vi "HTS_GET_PMC_COMMANDS.vi"(8 "Error IN":errorcluster, 11 "VISA resource IN":refnum<visa-resource-name>="HTS") -> (0 "Error OUT":errorcluster, 2 "HTS_PMC_COMMANDS":T1, 3 "VISA resource OUT":refnum<visa-resource-name>)   [LabVIEW 2009]
uses:
  HTS_PMC_COMMAND_LIST.ctl
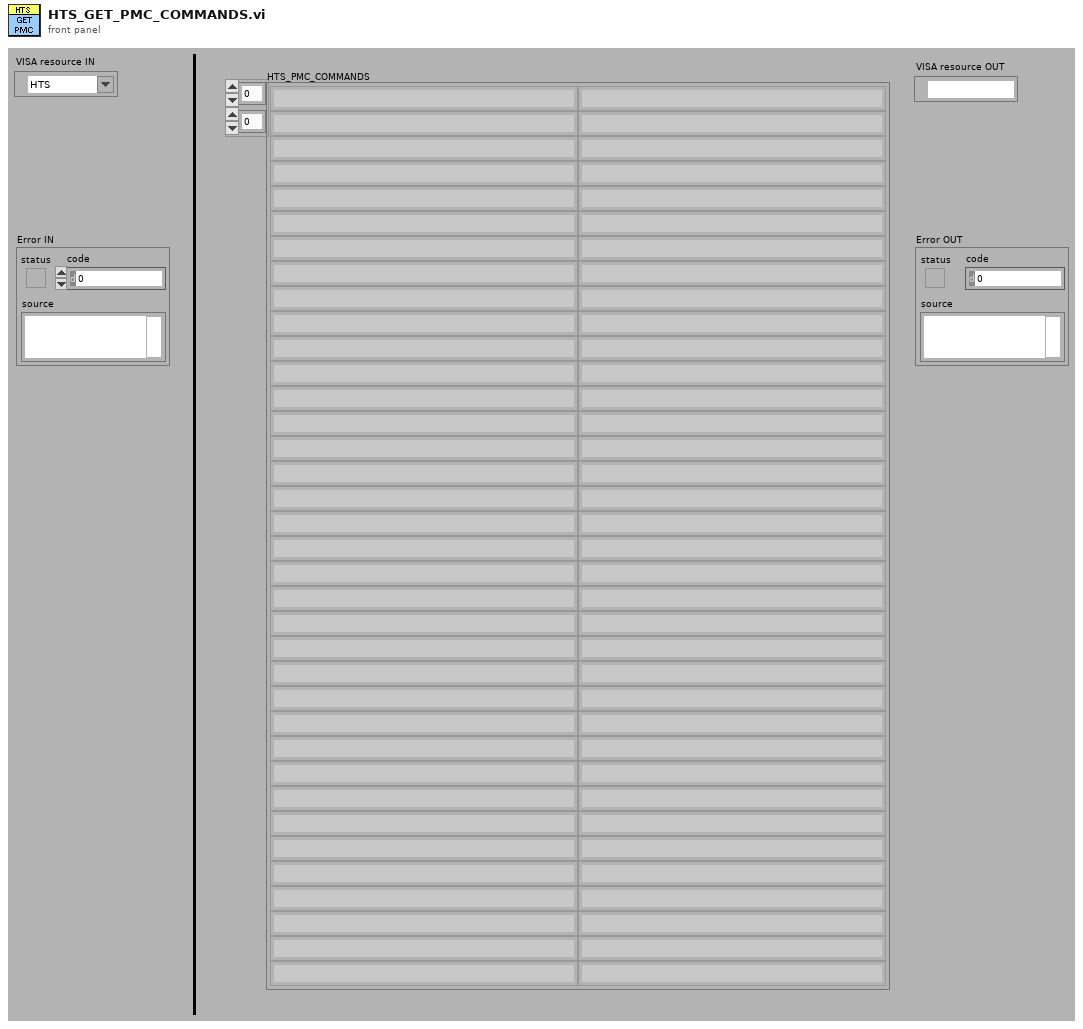
[diagram p1: front panel]
types:
  T1 = typedef "HTS_PMC_COMMAND_LIST.ctl" = string[][]
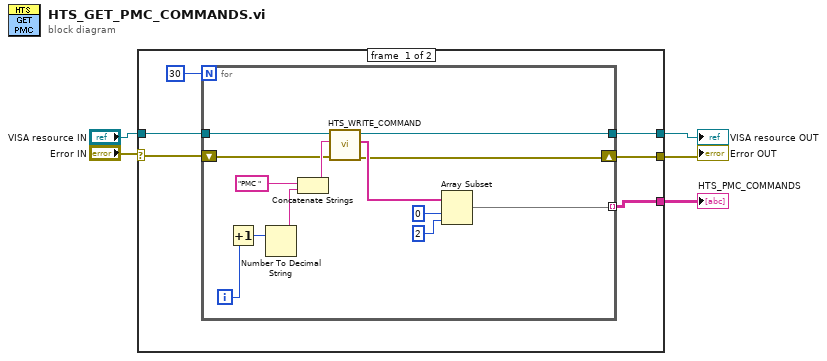
[diagram p0: block diagram]
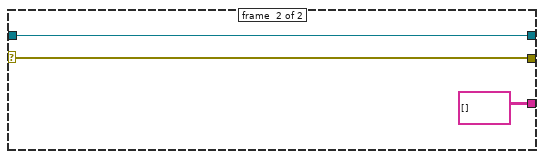
[diagram p2: hidden frame]
diagram:
  n1 = case shown="No Error" "Error IN" {
    selector: "Error IN" -> [w6 w26]
    tunnel: "VISA resource IN" -> [w11 w27]
    tunnel: [w9 string[][] []] -> w4
    tunnel: [w8 w26] -> w3
    tunnel: [w7 w27] -> w2
    frame #0 {
      n2 = for {
        N: 30 -> [_]
        tunnel: w11 -> [w24]
        tunnel: [w20] -> w9 mode=indexing
        shift-right: [w15] -> w8
        shift-left: w6 -> [w16]
        tunnel: [w12] -> w7
        i -> [w14]
        n3 = Increment(x=w14) -> (x+1=w13:i32)
        n4 = Number To Decimal String(number=w13) -> (decimal integer string=w19:string)  [unwired: 1 out]
        n5 = Concatenate Strings("PMC ", w19) -> (w17:string)
        n6 = call "HTS_WRITE_COMMAND.vi"("Error IN"=w16, "Command"=w17, "VISA resource IN"=w24) -> ("Error OUT"=w15:errorcluster, "RESPONSE"=w23:string[], "VISA resource OUT"=w12:refnum<visa-resource-name>)  [unwired: 6 out]
        n7 = Array Subset(array=w23, index=0, length=2) -> (w20:string[])
      }
    }
    frame #1 {
    }
  }
  "HTS_PMC_COMMANDS" <- w4
  "Error OUT" <- w3
  "VISA resource OUT" <- w2
